vi "D2SParser - Private - Function - Read Character Class.vi"(8 "error in (no error)":errorcluster, 11 "D2SParser in":refnum<class "D2SParser.lvclass">) -> (0 "error out":errorcluster, 3 "D2SParser out":refnum<class "D2SParser.lvclass">)   [LabVIEW 2015, in "D2SParser.lvclass"]
uses:
  D2SParser.lvclass
  D2SParser.lvclass/D2SParser.ctl
  D2Character/D2Character - Char Class.ctl
  D2Character/D2Character.lvclass/D2Character.ctl
  D2Character/D2Character - Accessors - Set Class.vi
  D2SParser - Private - Helper - Read Byte.vi
  D2SkillsTable/D2SkillsTable - Public - Functions - Build Table.vi
  D2Character/D2Character.lvclass
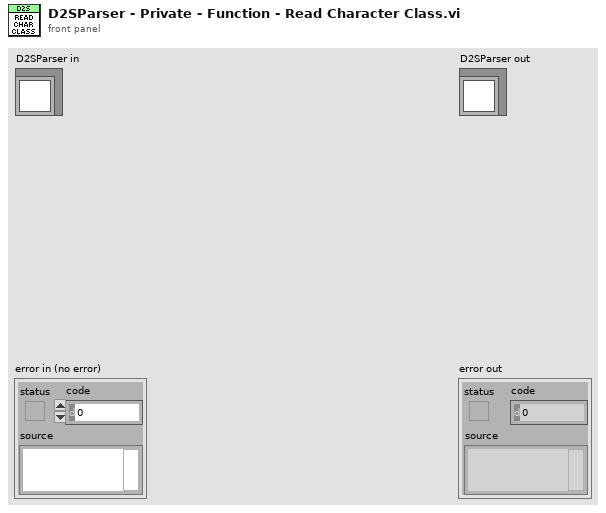
[diagram p1: front panel]
types:
  T1 = typedef "D2Character.lvclass/D2Character - Char Class.ctl" = enum8{"Amazon", "Sorceress", "Necromancer", "Paladin", "Barbarian", "Druid", "Assassin"}
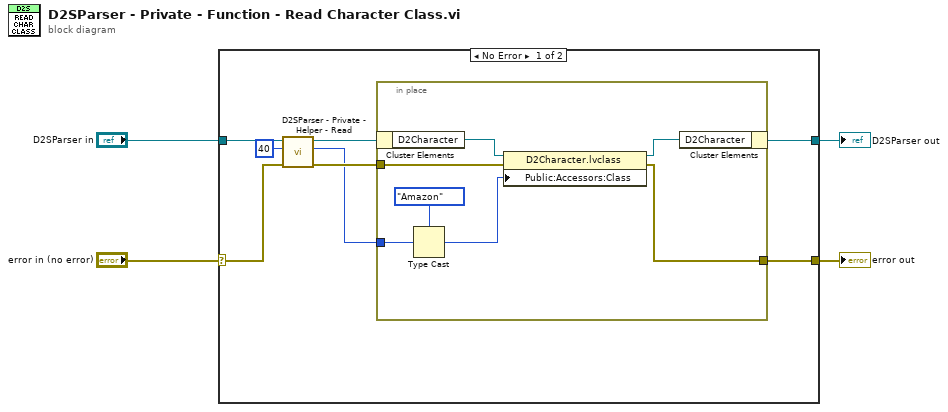
[diagram p0: block diagram]
diagram:
  n1 = case shown="No Error" "error in (no error)" {
    selector: "error in (no error)" -> [w11 w21]
    tunnel: [w8 w21] -> w3
    tunnel: [w7 w20] -> w1
    tunnel: "D2SParser in" -> [w12 w20]
    frame No Error {
      n2 = call-poly "D2SParser - Private - Helper - Read.vi"("error in (no error)"=w11, "Position"=i64 40, "D2SParser in"=w12) -> ("error out"=w9:errorcluster, "byte"=w5:u8, "D2SParser out"=w10:refnum<class "D2SParser.lvclass">)  [unwired: 6 in]
      n3 = in-place {
        in-place-border: w9 -> [w17]
        in-place-border: [w16] -> w8
        in-place-border: w5 -> [w15]
        n4 = in-place-cluster #1(w10) -> ("D2Character"=w19:refnum<class "D2Character.lvclass">)
        n5 = Type Cast(type=D2Character_-_Char_Class."Amazon" ("Class"), x=w15) -> (*(type *) &x=w13:T1)
        n6 = property class="D2Character.lvclass"(reference=w19, error in=w17, "Public:Accessors:Class"=w13) -> (reference out=w18:refnum<class "D2Character.lvclass">, error out=w16:errorcluster)
        n7 = in-place-cluster #1("D2Character"=w18) -> (w7:refnum<class "D2SParser.lvclass">)
      }
    }
    frame Error {
    }
  }
  "error out" <- w3
  "D2SParser out" <- w1
